vi "Get EDS Module Information.vi"(5 "Password":string, 7 "Username":string="admin", 8 "error in (no error)":errorcluster, 9 "Slot #":u32=4, 10 "Chassis IP Address":string, 11 "SLSC EDS System Tests in":refnum<class "SLSC EDS System Tests.lvclass">) -> (0 "error out":errorcluster, 3 "SLSC EDS System Tests out":refnum<class "SLSC EDS System Tests.lvclass">)   [LabVIEW 2019, in "SLSC EDS System Tests.lvclass"]
uses:
  SLSC EDS System Tests.lvclass
  SLSC EDS System Tests.lvclass/SLSC EDS System Tests.ctl
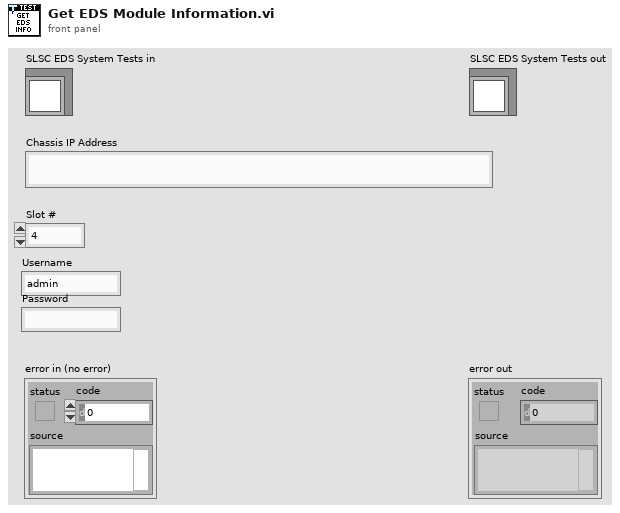
[diagram p1: front panel]
types:
  T1 = typedef "EDSjsonStructure.ctl" = cluster{"vendorNum":u32, "vendorName":string, "vendorPrefix":string, "productNum":u32, "productName":string, "capsVersion":string, "capsSpecVersion":u32, "capsSpecOldestCompatibleVersion":u32, "enums":T2[], "properties":T3[], "commands":T4[], "scales":T5[], "physicalChannels":T6[], "registerMap":cluster{"registers":T7[]}}
  T2 = typedef "enum.ctl" = cluster{"name":string, "description-en":string, "values":cluster{"name":string, "description-en":string, "value":i32}[]}
  T3 = typedef "property.ctl" = cluster{"name":string, "description-en":string, "documentation-en":string, "dataType":string, "bitfield":string, "access":string, "scale":string, "value":variant, "min":variant, "max":variant, "default value":variant}
  T4 = typedef "command.ctl" = cluster{"name":string, "description-en":string, "documentation-en":string, "startBitfield":string, "waitTimeInMs":i32, "doneBitfield":string, "doneInterrupt":string, "doneTimeoutInMs":i32, "value":variant}
  T5 = typedef "scale.ctl" = cluster{"name":string, "description-en":string, "m":dbl, "b":dbl, "forwardCoeffs":dbl[], "reverseCoeffs":dbl[], "coercion":string, "table":cluster{"scaled":dbl, "unscaled":dbl}[]}
  T6 = typedef "physicalChannel.ctl" = cluster{"name":string, "description-en":string, "commands":T4[], "properties":T3[]}
  T7 = typedef "register.ctl" = cluster{"name":string, "description-en":string, "access":string, "address":u32, "size":u32, "bitfields":cluster{"name":string, "description-en":string, "offset":u32, "size":u32, "signed":bool, "strobe":bool}[]}
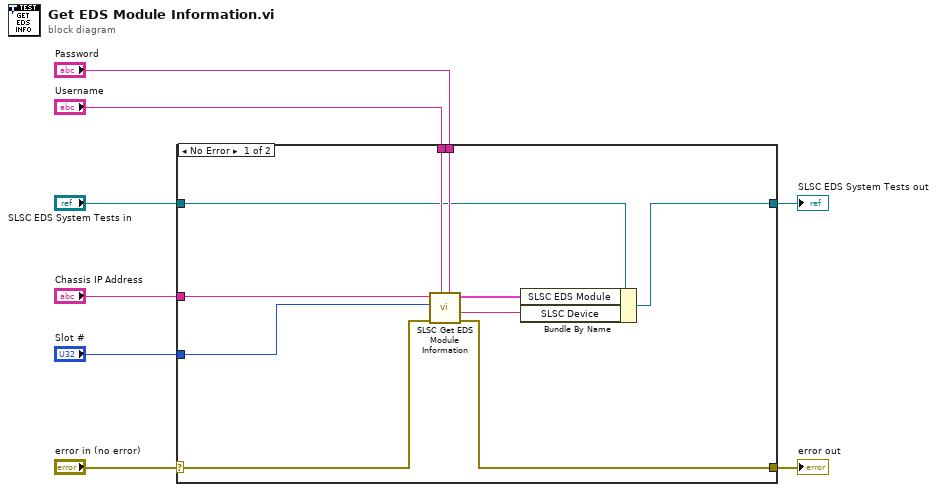
[diagram p0: block diagram]
diagram:
  n1 = case shown="No Error" "error in (no error)" {
    selector: "error in (no error)" -> [w18 w20]
    tunnel: [w17 w20] -> w7
    tunnel: [w12 w19] -> w5
    tunnel: "SLSC EDS System Tests in" -> [w9 w19]
    tunnel: "Chassis IP Address" -> [w16 _]
    tunnel: "Slot #" -> [w15 _]
    tunnel: "Username" -> [w11 _]
    tunnel: "Password" -> [w10 _]
    frame No Error {
      n2 = call "SLSC Get EDS Module Information.vi"("Password"=w10, "Username"=w11, "error in (no error)"=w18, "Slot #"=w15, "Chassis IP Address"=w16) -> ("error out"=w17:errorcluster, "SLSC Module Name"=w13:string, "SLSC EDS module"=w14:T1)  [unwired: 3 in, 1 out]
      n3 = Bundle By Name(cluster=w9, "SLSC EDS Module"=w14, "SLSC Device"=w13) -> (w12:refnum<class "SLSC EDS System Tests.lvclass">)
    }
    frame Error {
    }
  }
  "error out" <- w7
  "SLSC EDS System Tests out" <- w5
